vi "PutData.vi"(8 "error in":errorcluster, 9 "Value":u32, 10 "Location":u32, 11 "Port":refnum<visa-resource-name>) -> (0 "error out":errorcluster, 3 "Port out":refnum<visa-resource-name>)   [LabVIEW 2021]
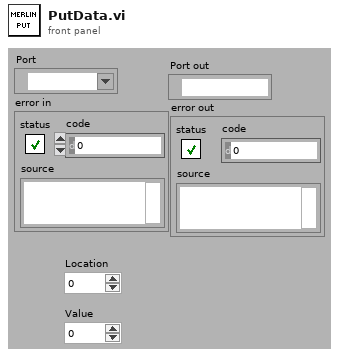
[diagram p1: front panel]
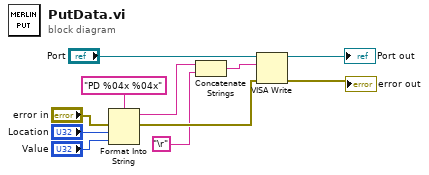
[diagram p0: block diagram]
diagram:
  n1 = Format Into String(format string="PD %04x %04x" ("concatenated string"), error in="error in", "Location", "Value") -> (resulting string=w10:string, error out=w8:errorcluster)  [unwired: 1 in]
  n2 = Concatenate Strings(w10, "\r") -> (w2:string)
  n3 = VISA Write(VISA resource name="Port", write buffer=w2, error in (no error)=w8) -> (VISA resource name out=→"Port out":refnum<visa-resource-name>, error out=→"error out":errorcluster)  [unwired: 1 out]
